vi "Test Control.vi"(10 "Command":T1=enum."Init") -> (1 "notifier out":refnum<notifier>)   [LabVIEW 2015]
uses:
  Test Control Command.ctl
  Sequence State Enum.ctl
  Clock Control Enum.ctl
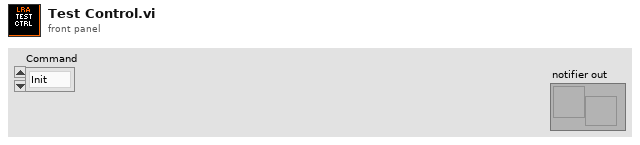
[diagram p1: front panel]
types:
  T1 = typedef "Test Control Command.ctl" = enum16{"Get Notifier", "Init", "Start", "Stop"}
  T2 = typedef "Clock Control Enum.ctl" = enum16{"Set", "Get", "Start", "Stop", "Sequence Init"}
  T3 = typedef "Sequence State Enum.ctl" = enum16{"Stopped", "Start", "Running", "Abort", "End"}
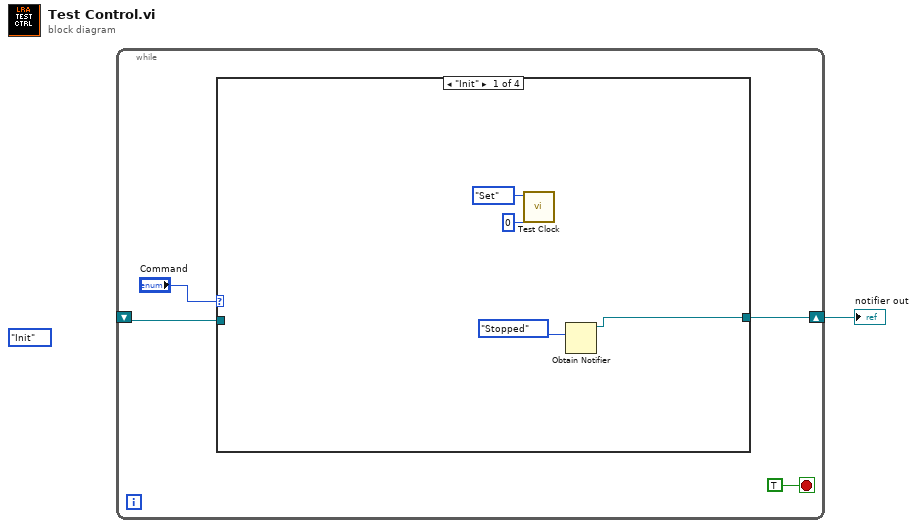
[diagram p0: block diagram]
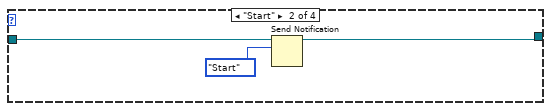
[diagram p2: hidden frame]
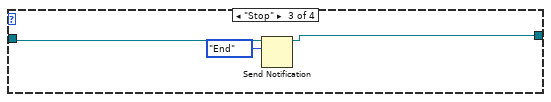
[diagram p3: hidden frame]
diagram:
  (unwired) Test_Control_Command."Init"
  n1 = while {
    shift-right: [w2] -> w1
    shift-left: _ -> [w3]
    stop <- TRUE stop-if-true
    n2 = case shown="\"Init\"" "Command" {
      tunnel: [w8 w10 w13 w16] -> w2
      tunnel: w3 -> [_ w12 w15 w16]
      frame "Init" {
        n3 = call "Test Clock.vi"("Set Time"=0, "Command"=Clock_Control_Enum."Set") -> ()  [unwired: 7 in, 3 out]
        n4 = Obtain Notifier(notification data type=Sequence_State_Enum."Stopped") -> (notifier out=w8:refnum<notifier>)  [unwired: 3 in, 2 out]
      }
      frame "Start" {
        n5 = Send Notification(notification=Sequence_State_Enum."Start", notifier=w12) -> (notifier out=w10:refnum<notifier>)  [unwired: 1 in, 1 out]
      }
      frame "Stop" {
        n6 = Send Notification(notification=Sequence_State_Enum."End", notifier=w15) -> (notifier out=w13:refnum<notifier>)  [unwired: 1 in, 1 out]
      }
      frame "Get Notifier" {
      }
    }
  }
  "notifier out" <- w1
